vi "VaisalaHMP60_SerialData.vi"(0 "Port Number":refnum<visa-resource-name>="COM1", 1 "Baud Rate":u32=19200, 6 "Save?":bool, 10 "File Name (dialog if empty)":path=path "C:/Users/BBCES/Desktop") -> (8 "T (C)":dbl, 9 "RH (%)":dbl)   [LabVIEW 2011]
doc: "The Basic Serial Read and Write example performs a Serial Port Read, a Serial Port Write, or a combination of these actions. The user selects the actions (read or write) on the front panel. If both are selected, the VI will write the data first, read data, and then close the VISA session that is opened to the port. This VI will wait until the specified number of bytes is received at the port or until a termination character is read.\n\nINSTRUCTIONS:\n1) Select the serial resource and configuration parameters (baud rate, data bits, parity, stop bits, flow control).\n2) Select the operations to be performed. \n3) Connect the serial port to your device. If no device is available, perform a loopback test by doing one of the following. Short pins 2 and 3 on a RS-232 cable or short pin 4 to pin 8 and pin 5 to pin 9 on a RS-485/422 cable. \n4) Run the VI to see the data read. (The \"read string\" will match the \"string to write\" if a loopback test was performed.)\n\nNote: The parameters set for the serial port must match the parameters of the connected instrument or device. In this example, the bytes to read parameter specifies the number of bytes that the serial port reads. If there were more bytes at the port than the number specified in bytes to read, those bytes would not be read. Also, if you specify to read more bytes than the number of bytes actually read, you might receive a timeout error message.\n\nOn the block diagram, the Configure Serial Port VI sets the configuration parameters. The front panel displays the controls used to configure the basic parameters, such as baud rate, data bits, and parity. Constants configure the other parameters the user probably does not need set. After the VISA Configure Serial Port VI opens the VISA session and configures the port, the VI passes the VISA resource name to other VIs that perform operations on that VISA resource. The VISA Write function sends a command to the serial device and the VISA Read function returns data based on the command. The VISA Close function then closes the reference to the serial device. It is important to close the reference; otherwise communication through with that port through protocols other than VISA might not be possible."
uses:
  <vilib>/Instr/_visa.llb/VISA Configure Serial Port (Instr).vi
  <vilib>/Utility/file.llb/Write To Spreadsheet File (string).vi
panel:
  out "Relative Humidity":dbl[](graph)
  out "Temperature":dbl[](graph)
  out "Dp (C)":dbl
  in  "stop":bool
  # "Instructions:\n\n1.  Connect the Vaisala USB cable but DO NOT connect the probe to the cable.\n2.  Open PuTTY and select the correct COM port.  The default values are:\n            - Baud: 19200\n            - Data bits: 8\n            - Stop bits: 1\n            - Parity: None\n            - Flow Control: None\n3.  Click \"Open\".\n4.  While holding down the \"Enter\" key, connect the probe to the cable.  This initializes the probe in RS-485 mode.\n5.  Close the PuTTY window and confirm closing the session.\n6.  Begin collecting data with LabVIEW."
  # "Vaisala HMP60 Serial Data Interface"
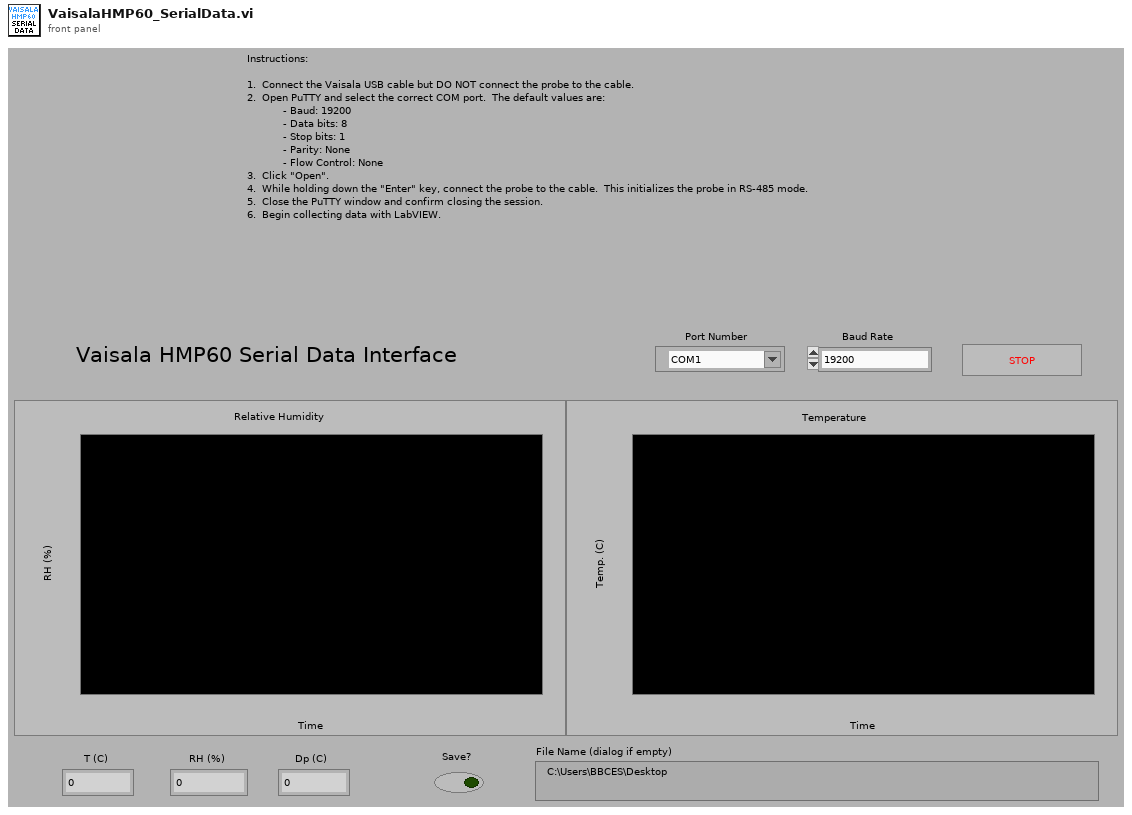
[diagram p1: front panel]
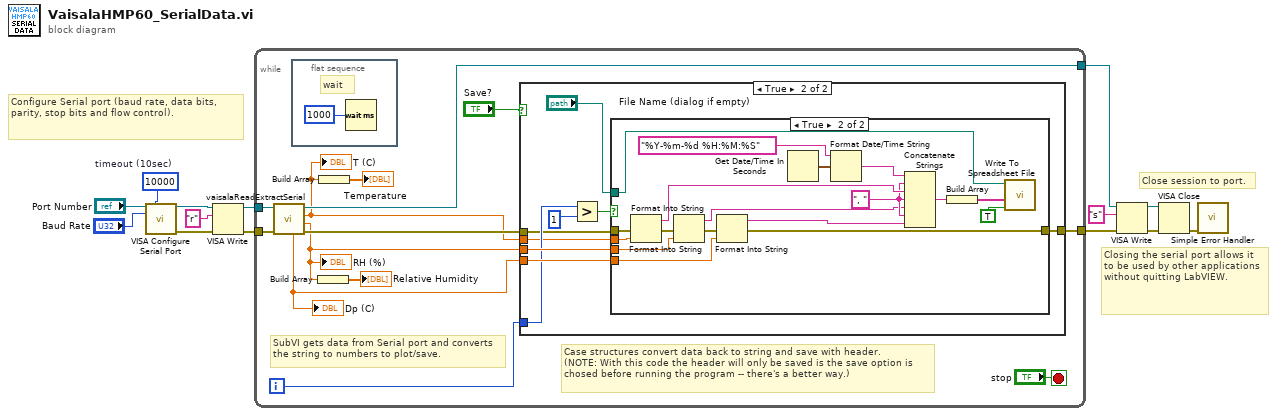
[diagram p0: block diagram]
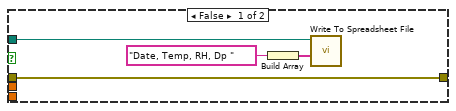
[diagram p3: hidden frame]
diagram:
  w11 = u32 10000  # timeout (10sec)
  # "Closing the serial port allows it to be used by other applications without quitting LabVIEW."
  # "Configure Serial port (baud rate, data bits, parity, stop bits and flow control)."
  # "Close session to port."
  n1 = call-poly "VISA Configure Serial Port"("VISA resource name"="Port Number", "timeout (10sec)"=w11, "baud rate (9600)"="Baud Rate") -> ("VISA resource name out"=w1:refnum<visa-resource-name>, "error out"=w2:errorcluster)  [unwired: 6 in, 5 out]
  n2 = VISA Write(VISA resource name=w1, write buffer="r", error in (no error)=w2) -> (VISA resource name out=w9:refnum<visa-resource-name>, error out=w10:errorcluster)  [unwired: 1 out]
  n3 = while {
    tunnel: [w20] -> w6
    tunnel: [w26] -> w7
    tunnel: w10 -> [w25]
    tunnel: w9 -> [w24]
    i -> [w19]
    stop <- "stop" stop-if-true
    # "Case structures convert data back to string and save with header.\n(NOTE: With this code the header will only be saved is the save option is chosed before running the program -- there's a better way.)"
    # "SubVI gets data from Serial port and converts the string to numbers to plot/save."
    n4 = call "vaisalaReadExtractSerial.vi"("error in (no error)"=w25, "VISA Refnum in"=w24) -> ("error out"=w21:errorcluster, "RH (%)"=w17:dbl, "T (C)"=w15:dbl, "VISA Refnum out"=w26:refnum<visa-resource-name>, "Dp (C)"=w18:dbl)  [unwired: 5 in]
    "T (C)" <- w15
    "RH (%)" <- w17
    "Dp (C)" <- w18
    n5 = flat-sequence {
      frame #0 {
        # "wait"
        n6 = Wait (ms)(milliseconds to wait=u32 1000) -> ()  [unwired: 1 out]
      }
    }
    n7 = Build Array(w17) -> (→"Relative Humidity":dbl[])
    n8 = Build Array(w15) -> (→"Temperature":dbl[])
    n9 = case shown="True" "Save?" {
      tunnel: w21 -> [w28 w30]
      tunnel: [w28 w36] -> w20
      tunnel: w17 -> [_ w37]
      tunnel: w18 -> [_ w35]
      tunnel: w19 -> [_ w31]
      tunnel: w15 -> [_ w29]
      frame False {
      }
      frame True {
        n10 = Greater?(x=w31, y=1) -> (0:w33:bool)
        n11 = case shown="True" w33 {
          tunnel: w37 -> [_ w53]
          tunnel: [w41 w50] -> w36
          tunnel: w35 -> [_ w49]
          tunnel: "File Name (dialog if empty)" -> [w38 w44]
          tunnel: w30 -> [w41 w43]
          tunnel: w29 -> [_ w42]
          frame False {
            n12 = Build Array("Date, Temp, RH, Dp " ("string")) -> (w39:string[])
            n13 = call-poly <vilib>:"Write To Spreadsheet File.vi"("1D data"=w39, "file path (dialog if empty)"=w38) -> ()  [unwired: 6 in, 1 out]
          }
          frame True {
            w47 = ", " ("string")
            n14 = Format Into String(error in=w43, w42) -> (resulting string=w48:string, error out=w52:errorcluster)  [unwired: 2 in]
            n15 = Format Into String(error in=w52, w53) -> (resulting string=w46:string, error out=w51:errorcluster)  [unwired: 2 in]
            n16 = Format Into String(error in=w51, w49) -> (resulting string=w45:string, error out=w50:errorcluster)  [unwired: 2 in]
            n17 = Get Date/Time In Seconds() -> (seconds since 1Jan1904=w58:timestamp)
            n18 = Format Date/Time String(time format string (%c)="%Y-%m-%d %H:%M:%S", seconds (now)=w58) -> (date/time string=w57:string)  [unwired: 1 in]
            n19 = Concatenate Strings(w57, w47, w48, w47, w46, w47, w45) -> (w56:string)
            n20 = Build Array(w56) -> (w55:string[])
            n21 = call-poly <vilib>:"Write To Spreadsheet File.vi"("append to file? (new file:F)"=TRUE, "1D data"=w55, "file path (dialog if empty)"=w44) -> ()  [unwired: 5 in, 1 out]
          }
        }
      }
    }
  }
  n22 = VISA Write(VISA resource name=w7, write buffer="s", error in (no error)=w6) -> (VISA resource name out=w5:refnum<visa-resource-name>, error out=w4:errorcluster)  [unwired: 1 out]
  n23 = VISA Close(VISA resource name=w5, error in (no error)=w4) -> (error out=w12:errorcluster)
  n24 = call <vilib>:"Simple Error Handler.vi"("error in (no error)"=w12) -> ()  [unwired: 1 in, 8 out]
